vi "TSM Set DAQmx Tasks.vi"(0 "TSM context":T1) -> (15 "error out":errorcluster)   [LabVIEW 2020]
doc: "Use this VI to initialize AI and AO tasks for all NI-DAQmx instruments in the pin map associated with the test program."
uses:
  <vilib>/NI_TestStand_SemiconductorModule/NI_TestStand_Semiconductor_Module.lvlibp/PinMap/General/SemiconductorModuleContext.ctl
  <vilib>/NI_TestStand_SemiconductorModule/NI_TestStand_Semiconductor_Module.lvlibp
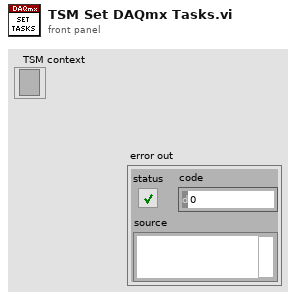
[diagram p1: front panel]
types:
  T1 = typedef "NI_TestStand_Semiconductor_Module.lvlibp/SemiconductorModuleContext.ctl" = refnum<k7>
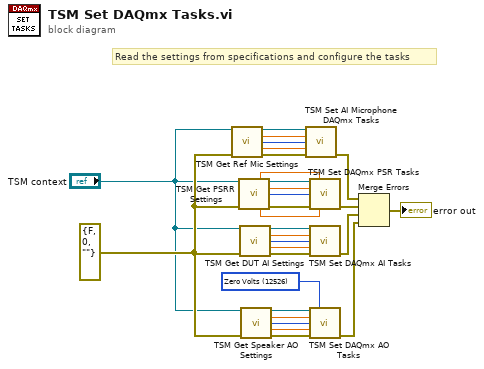
[diagram p0: block diagram]
diagram:
  w1 = 12526 items=["Zero Volts"=12526, "High-Impedance"=12527, "Maintain Existing Value"=12528] ("IdleOutputBehavior (Zero Volts)")
  w8 = errorcluster {"status"=FALSE, "code"=0, "source"=""} ("error in (no error)")
  # "Read the settings from specifications and configure the tasks"
  n1 = call "TSM Get Ref Mic Settings.vi"("TSM context"="TSM context", "error in (no error)"=w8) -> ("TSM context Out"=w23:T1, "Sampling Rate (Hz)"=w22:dbl, "Samples per channel"=w21:i32, "max dB SPL"=w20:dbl, "error out"=w24:errorcluster)  [unwired: 8 in, 1 out]
  n2 = call "TSM Get PSRR Settings.vi"("TSM context"="TSM context", "error in (no error)"=w8) -> ("max V"=w17:dbl, "TSM context Out"=w19:T1, "Sampling Rate (Hz)"=w15:dbl, "Samples per channel"=w14:i32, "min V"=w16:dbl, "error out"=w18:errorcluster)  [unwired: 8 in]
  n3 = call "TSM Get DUT AI Settings.vi"("TSM context"="TSM context", "error in (no error)"=w8) -> ("TSM context Out"=w13:T1, "Sampling Rate (Hz)"=w11:dbl, "Samples per channel"=w10:i32, "Range (V)"=w9:dbl, "error out"=w12:errorcluster)  [unwired: 9 in]
  n4 = call "TSM Get Speaker AO Settings.vi"("TSM context"="TSM context", "error in (no error)"=w8) -> ("TSM context Out"=w6:T1, "Sampling Rate (Hz)"=w4:dbl, "Samples per channel"=w3:i32, "Range (V)"=w2:dbl, "error out"=w5:errorcluster)  [unwired: 9 in]
  n5 = call "TSM Set AI Microphone DAQmx Tasks.vi"("TSM context"=w23, "Sampling Rate (Hz)"=w22, "Samples per channel"=w21, "max dB SPL"=w20, "error in (no error)"=w24) -> ("error out"=w28:errorcluster)  [unwired: 10 in]
  n6 = call "TSM Set DAQmx PSR Tasks.vi"("TSM context"=w19, "max V"=w17, "Sampling Rate (Hz)"=w15, "samples per channel"=w14, "error in (no error)"=w18, "min V"=w16) -> ("error out"=w27:errorcluster)  [unwired: 9 in]
  n7 = call "TSM Set DAQmx AI Tasks.vi"("TSM context"=w13, "Sampling Rate (Hz)"=w11, "Samples per channel"=w10, "Range (V)"=w9, "error in (no error)"=w12) -> ("error out"=w26:errorcluster)  [unwired: 10 in]
  n8 = call "TSM Set DAQmx AO Tasks.vi"("TSM context"=w6, "IdleOutputBehavior (Zero Volts)"=w1, "Sampling Rate (Hz)"=w4, "Samples per channel"=w3, "Range (V)"=w2, "error in (no error)"=w5) -> ("error out"=w25:errorcluster)  [unwired: 9 in]
  n9 = Merge Errors(w28, w27, w26, w25) -> (→"error out":errorcluster)
